vi "Main Rufus.vi"() -> ()   [LabVIEW 2017]
uses:
  Raw Oculus Data.ctl
  Calibrated Oculus Data.ctl
  <extravilib>/ChannelInstances/Lossy Stream-t'Calibrated Oculus Data.ctl'/Read With Abort.vi
  <extravilib>/ChannelInstances/Lossy Stream-t'Calibrated Oculus Data.ctl'/Write With Abort.vi
  <extravilib>/ChannelInstances/Lossy Stream-t'Calibrated Oculus Data.ctl'/EndpointRead.vi
  <extravilib>/ChannelInstances/Lossy Stream-t'Calibrated Oculus Data.ctl'/Endpoint.vi
  <extravilib>/ChannelInstances/Lossy Stream-t'Calibrated Oculus Data.ctl'/Instantiate.vi
  <extravilib>/ChannelInstances/Lossy Stream-t'Calibrated Oculus Data.ctl'/)Channel.vi
  <resource>/ChannelSupport/_ChannelSupport/WaitIfNeeded.vi
  <extravilib>/ChannelInstances/Lossy Stream-t'Calibrated Oculus Data.ctl'.lvlib
panel:
  in  "Hold head":bool
  out "Calibration Complete":bool
  out "error out":errorcluster
  out "uArm read buffer":string
  out "Calibrated Oculus Data":T1
  out "Raw Oculus Data":T2
  in  "Boundary":T3={"X max"=310.0, "X min"=147.0, "Z max"=148.0, "Z min"=-92.0}
  in  "VISA Refnum in":refnum<visa-resource-name>="ASRL3::INSTR"
  in  "error in":errorcluster
  in  "Arm X Max":dbl=340.0
  in  "Arm X Min":dbl=90.0
  # "START PROCEDURE\nMake sure the arm max and min are set to the correct\nvalues. Keep them just off the boundaries for the best \nresults\n1 - Press A to set your hand's origin position\n2 - Press B to set your hand's maximum X position\n3 - Press X to set the calibration and start sending data\n   - Before step 3 you may repeate steps 1 and 2 as much\n      as you'd like. After hitting X however the calibration\n      is set.\n4 - Press Menu to end this program (or the stop button on\n      the front pannel) at any time\n\nCONTROLS AFTER START\nThe Uarm will follow your right hand as best it can, Move slow though.\n\nA - Hold current Z position.\nB - Hold current wrist angle.\nSqueeze Right Trigger - Close Grippers\nRelease Right Trigger - Release Grippers\nMenu - Exit program"
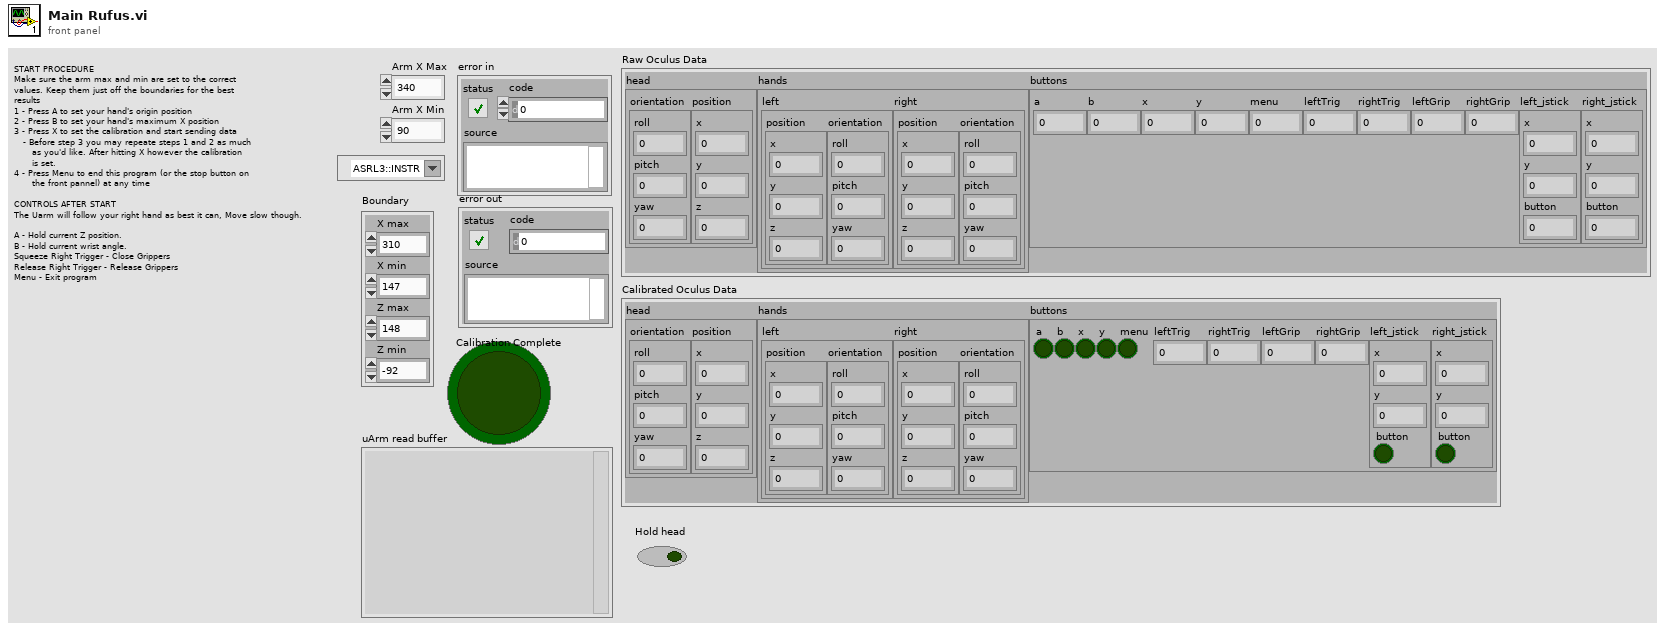
[diagram p1: front panel]
types:
  T1 = typedef "Calibrated Oculus Data.ctl" = cluster{"head":cluster{"orientation":cluster{"roll":dbl, "pitch":dbl, "yaw":dbl}, "position":cluster{"x":dbl, "y":dbl, "z":dbl}}, "hands":cluster{"left":cluster{"position":cluster{"x":dbl, "y":dbl, "z":dbl}, "orientation":cluster{"roll":dbl, "pitch":dbl, "yaw":dbl}}, "right":cluster{"position":cluster{"x":dbl, "y":dbl, "z":dbl}, "orientation":cluster{"roll":dbl, "pitch":dbl, "yaw":dbl}}}, "buttons":cluster{"a":bool, "b":bool, "x":bool, "y":bool, "menu":bool, "leftTrig":dbl, "rightTrig":dbl, "leftGrip":dbl, "rightGrip":dbl, "left_jstick":cluster{"x":dbl, "y":dbl, "button":bool}, "right_jstick":cluster{"x":dbl, "y":dbl, "button":bool}}}
  T2 = typedef "Raw Oculus Data.ctl" = cluster{"head":cluster{"orientation":cluster{"roll":dbl, "pitch":dbl, "yaw":dbl}, "position":cluster{"x":dbl, "y":dbl, "z":dbl}}, "hands":cluster{"left":cluster{"position":cluster{"x":dbl, "y":dbl, "z":dbl}, "orientation":cluster{"roll":dbl, "pitch":dbl, "yaw":dbl}}, "right":cluster{"position":cluster{"x":dbl, "y":dbl, "z":dbl}, "orientation":cluster{"roll":dbl, "pitch":dbl, "yaw":dbl}}}, "buttons":cluster{"a":i32, "b":i32, "x":i32, "y":i32, "menu":i32, "leftTrig":dbl, "rightTrig":dbl, "leftGrip":dbl, "rightGrip":dbl, "left_jstick":cluster{"x":dbl, "y":dbl, "button":i32}, "right_jstick":cluster{"x":dbl, "y":dbl, "button":i32}}}
  T3 = cluster{"X max":dbl, "X min":dbl, "Z max":dbl, "Z min":dbl}
  T4 = cluster{"left":cluster{"Center":cluster{"x":dbl, "y":dbl, "z":dbl}, "Max":dbl}, "right":cluster{"Center":cluster{"x":dbl, "y":dbl, "z":dbl}, "Max":dbl}}
  T5 = typedef "Lossy Stream-t'Calibrated Oculus Data.ctl'.lvlib/)Channel.ctl" = refnum<queue>
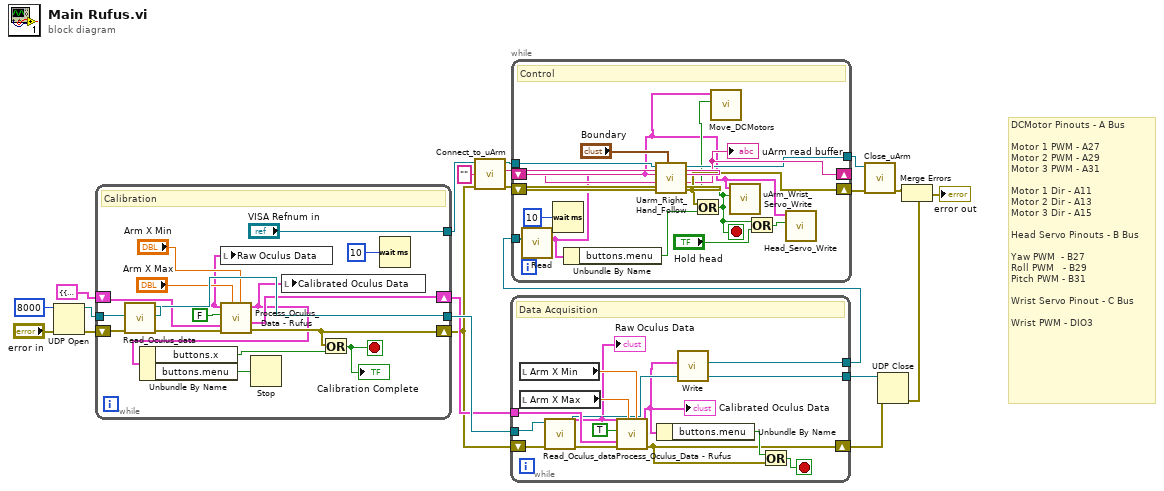
[diagram p0: block diagram]
diagram:
  # "DCMotor Pinouts - A Bus\n\nMotor 1 PWM - A27\nMotor 2 PWM - A29\nMotor 3 PWM - A31\n\nMotor 1 Dir - A11\nMotor 2 Dir - A13\nMotor 3 Dir - A15\n\nHead Servo Pinouts - B Bus\n\nYaw PWM  - B27\nRoll PWM   - B29\nPitch PWM - B31\n\nWrist Servo Pinout - C Bus\n\nWrist PWM - DIO3"
  n1 = UDP Open(8:"error in", 11:u16 8000 ("port")) -> (port=w20:refnum<k16>, 0:w21:errorcluster)  [unwired: 3 in, 1 out]
  n2 = while "Calibration" {
    tunnel: w20 -> [w37]
    tunnel: [w36] -> w17
    shift-right: [w30] -> w13
    shift-left: w21 -> [w38]
    tunnel: ["VISA Refnum in"] -> w15
    shift-right: [w28] -> w14
    shift-left: T4 {"left"={"Center"={"x"=0.0, "y"=0.0, "z"=0.0}, "Max"=0.0}, "right"={"Center"={"x"=0.0, "y"=0.0, "z"=0.0}, "Max"=0.0}} ("Calibration Data out") -> [w29]
    stop <- w34 stop-if-true
    # "Calibration"
    n3 = call "Read_Oculus_data.vi"("error in (no error)"=w38, "UDP Network Connection in"=w37) -> ("error out"=w31:errorcluster, "Raw Oculus Data"=w25:T2, "UDP Network Connection out"=w36:refnum<k16>)  [unwired: 7 in]
    n4 = local write "Raw Oculus Data"(w25) -> ()
    n5 = call "Process_Oculus_Data - Rufus.vi"("Arm X Min"="Arm X Min", "Arm X Max"="Arm X Max", "error in"=w31, "Calibration Data in"=w29, "Calibrated"=FALSE, "Raw Oculus Data"=w25) -> ("error out"=w30:errorcluster, "Calibration Data out"=w28:T4, "Calibrated Oculus Data"=w23:T1)  [unwired: 3 in]
    n6 = Unbundle By Name(w23) -> ("buttons.x"=w32:bool, "buttons.menu"=w24:bool)
    n7 = Stop(stop? (T)=w24) -> ()
    n8 = local write "Calibrated Oculus Data"(w23) -> ()
    n9 = Or(x=w32, y=w30) -> (x .or. y?=w34:bool)
    "Calibration Complete" <- w34
    n10 = Wait (ms)(milliseconds to wait=u32 10) -> ()  [unwired: 1 out]
  }
  n11 = call "Connect_to_uArm.vi"("error in"=w13, "full read buffer in"="", "Machine In"=w15) -> ("error out"=w6:errorcluster, "full read buffer out"=w5:string, "Machine Out"=w7:refnum<visa-resource-name>)  [unwired: 6 in]
  n12 = while "Data Aquisition" {
    shift-right: [w50] -> w18
    shift-left: w13 -> [w45]
    tunnel: w17 -> [w46]
    tunnel: [w43] -> w16
    tunnel: w14 -> [w51]
    tunnel: [w40] -> w4
    stop <- w47 stop-if-true
    # "Data Acquisition"
    n13 = local read "Arm X Min"() -> (w49:dbl)
    n14 = local read "Arm X Max"() -> (w48:dbl)
    n15 = call "Read_Oculus_data.vi"("error in (no error)"=w45, "UDP Network Connection in"=w46) -> ("error out"=w44:errorcluster, "Raw Oculus Data"=w42:T2, "UDP Network Connection out"=w43:refnum<k16>)  [unwired: 7 in]
    "Raw Oculus Data" <- w42
    n16 = call "Process_Oculus_Data - Rufus.vi"("Arm X Min"=w49, "Arm X Max"=w48, "error in"=w44, "Calibration Data in"=w51, "Calibrated"=TRUE, "Raw Oculus Data"=w42) -> ("error out"=w50:errorcluster, "Calibrated Oculus Data"=w39:T1)  [unwired: 3 in, 1 out]
    "Calibrated Oculus Data" <- w39
    n17 = Unbundle By Name(w39) -> ("buttons.menu"=w52:bool)
    n18 = call <extravilib>:"Write.vi"("element"=w39) -> ("channel"=w40:T5)  [unwired: 8 in, 2 out]
    n19 = Or(x=w52, y=w50) -> (x .or. y?=w47:bool)
  }
  n20 = while "Arm Control" {
    shift-right: [w62] -> _
    shift-left: w5 -> [w64]
    shift-right: [w63] -> w12
    shift-left: w6 -> [w58]
    tunnel: w4 -> [w54]
    tunnel: [w56] -> w11
    tunnel: w7 -> [w61]
    stop <- w55 stop-if-true
    # "Control"
    n21 = call <extravilib>:"Read.vi"("channel"=w54) -> ("element"=w53:T1)  [unwired: 5 in, 5 out]
    n22 = Wait (ms)(milliseconds to wait=u32 10) -> ()  [unwired: 1 out]
    n23 = Unbundle By Name(w53) -> ("buttons.menu"=w65:bool)
    n24 = call "Uarm_Right_Hand_Follow.vi"("Boundary"="Boundary", "error in"=w58, "full read buffer in"=w64, "Calibrated Oculus Data"=w53, "Machine In"=w61) -> ("error out"=w63:errorcluster, "full read buffer out"=w62:string, "Machine Out"=w56:refnum<visa-resource-name>)  [unwired: 4 in]
    "uArm read buffer" <- w62
    n25 = Or(x=w63, y=w65) -> (x .or. y?=w55:bool)
    n26 = call "Move_DCMotors.vi"("Stop"=w55, "Calibrated Oculus Data"=w53) -> ()  [unwired: 10 in]
    n27 = call "uArm_Wrist_Servo_Write.vi"("Stop"=w55, "Calibrated Oculus Data"=w53) -> ()  [unwired: 9 in, 1 out]
    n28 = Or(x=w55, y="Hold head") -> (x .or. y?=w59:bool)
    n29 = call "Head_Servo_Write.vi"("Stop"=w59, "Calibrated Oculus Data"=w53) -> ()  [unwired: 10 in]
  }
  n30 = call "Close_uArm.vi"("error in"=w12, "VISA Refnum in"=w11) -> ("error out"=w10:errorcluster)  [unwired: 9 in]
  n31 = UDP Close(connection ID=w16, 8:w18) -> (error out=w3:errorcluster)  [unwired: 1 out]
  n32 = Merge Errors(w10, w3) -> (→"error out":errorcluster)
